vi "TrigBasicType.vi"(3 "error in (no error)":errorcluster, 5 "task in":refnum<k24>) -> (0 "error out":errorcluster, 1 "TrigType":i32, 2 "task out":refnum<k24>)   [LabVIEW 2010]
uses:
  C:/Program Files/National Instruments/LabVIEW 2010/vi.lib/ULx/ULx_LV.dll
  Program Files/National Instruments/LabVIEW 2010/vi.lib/ULx/ULx_LV.dll
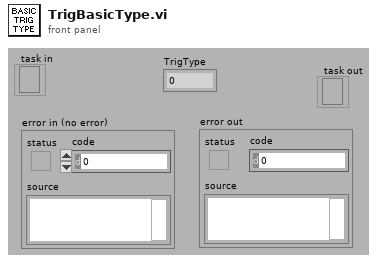
[diagram p1: front panel]
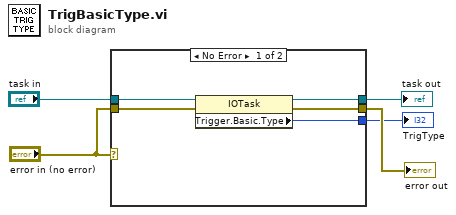
[diagram p0: block diagram]
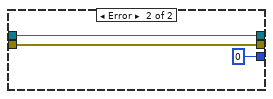
[diagram p2: hidden frame]
diagram:
  n1 = case shown="No Error" "error in (no error)" {
    tunnel: "task in" -> [w10 w13]
    tunnel: "error in (no error)" -> [w8 w12]
    tunnel: [w9 w13] -> w4
    tunnel: [w7 w12] -> w3
    tunnel: [w6 0 ("Trigger.Basic.Type")] -> w1
    frame No Error {
      n2 = property class="IOTask"(reference=w10, error in=w8) -> (reference out=w9:refnum<k24>, error out=w7:errorcluster, "Trigger.Basic.Type"=w6:i32)
    }
    frame Error {
    }
  }
  "task out" <- w4
  "error out" <- w3
  "TrigType" <- w1
